vi "Generate Signal.vi"(11 "User Specified":T1={"Hardware Configuration"={"Signal Channel"="PXI1Slot7/ao0", "Response Channel"="PXI1Slot7/ai0", "Trigger Channel"="/PXI1Slot7/PFI0", "Number of Acquisitions"=1.0}, "Analysis Configuration"={"Statistics"=TRUE}, "Signal Type"=enum."From Excel", "New Data Behavior"=enum."Replace", "Signal Configuration"={"Chirp Amplitude"=0.0, "I/O Limit"=0.0, "Sample Rate"=0.0, "Chirp Duration (s)"=0.0, "Upper Frequency"=0.0, "Lower Frequency"=0.0, "Windowing"=enum."None"}, "Waveform File"="", "Save Location"=""}) -> (0 "Number of samples":dbl format="%0.2f", 1 "Y min":dbl format="%0.2f", 2 "Y max":dbl format="%0.2f", 3 "Final Waveform":waveform(dbl)(graph))   [LabVIEW 2017]
uses:
  controls/User Specified Data.ctl
  controls/HW Configuration.ctl
  controls/Analysis Configuration.ctl
  controls/New Data Behavior.ctl
  controls/Signal Configuration.ctl
  <vilib>/Waveform/WDTOps.llb/WDT Append Waveforms DBL.vi
  <vilib>/Waveform/WDTOps.llb/WDT Number of Waveform Samples DBL.vi
panel:
  out "Initial waveform":waveform(dbl)
  out "Shift register waveform":waveform(dbl)(graph)
  out "Number of rows":i32
  out "Voltage Offset":dbl
  out "Single Chirp w/ offset":waveform(dbl)(graph)
  out "Samples per chirp":dbl
  out "Single Chirp (Excel)":waveform(dbl)(graph)
  out "error out":errorcluster
  in  "error in":errorcluster
  # "D:\\Data\\7-02-2018\\SSPFM"
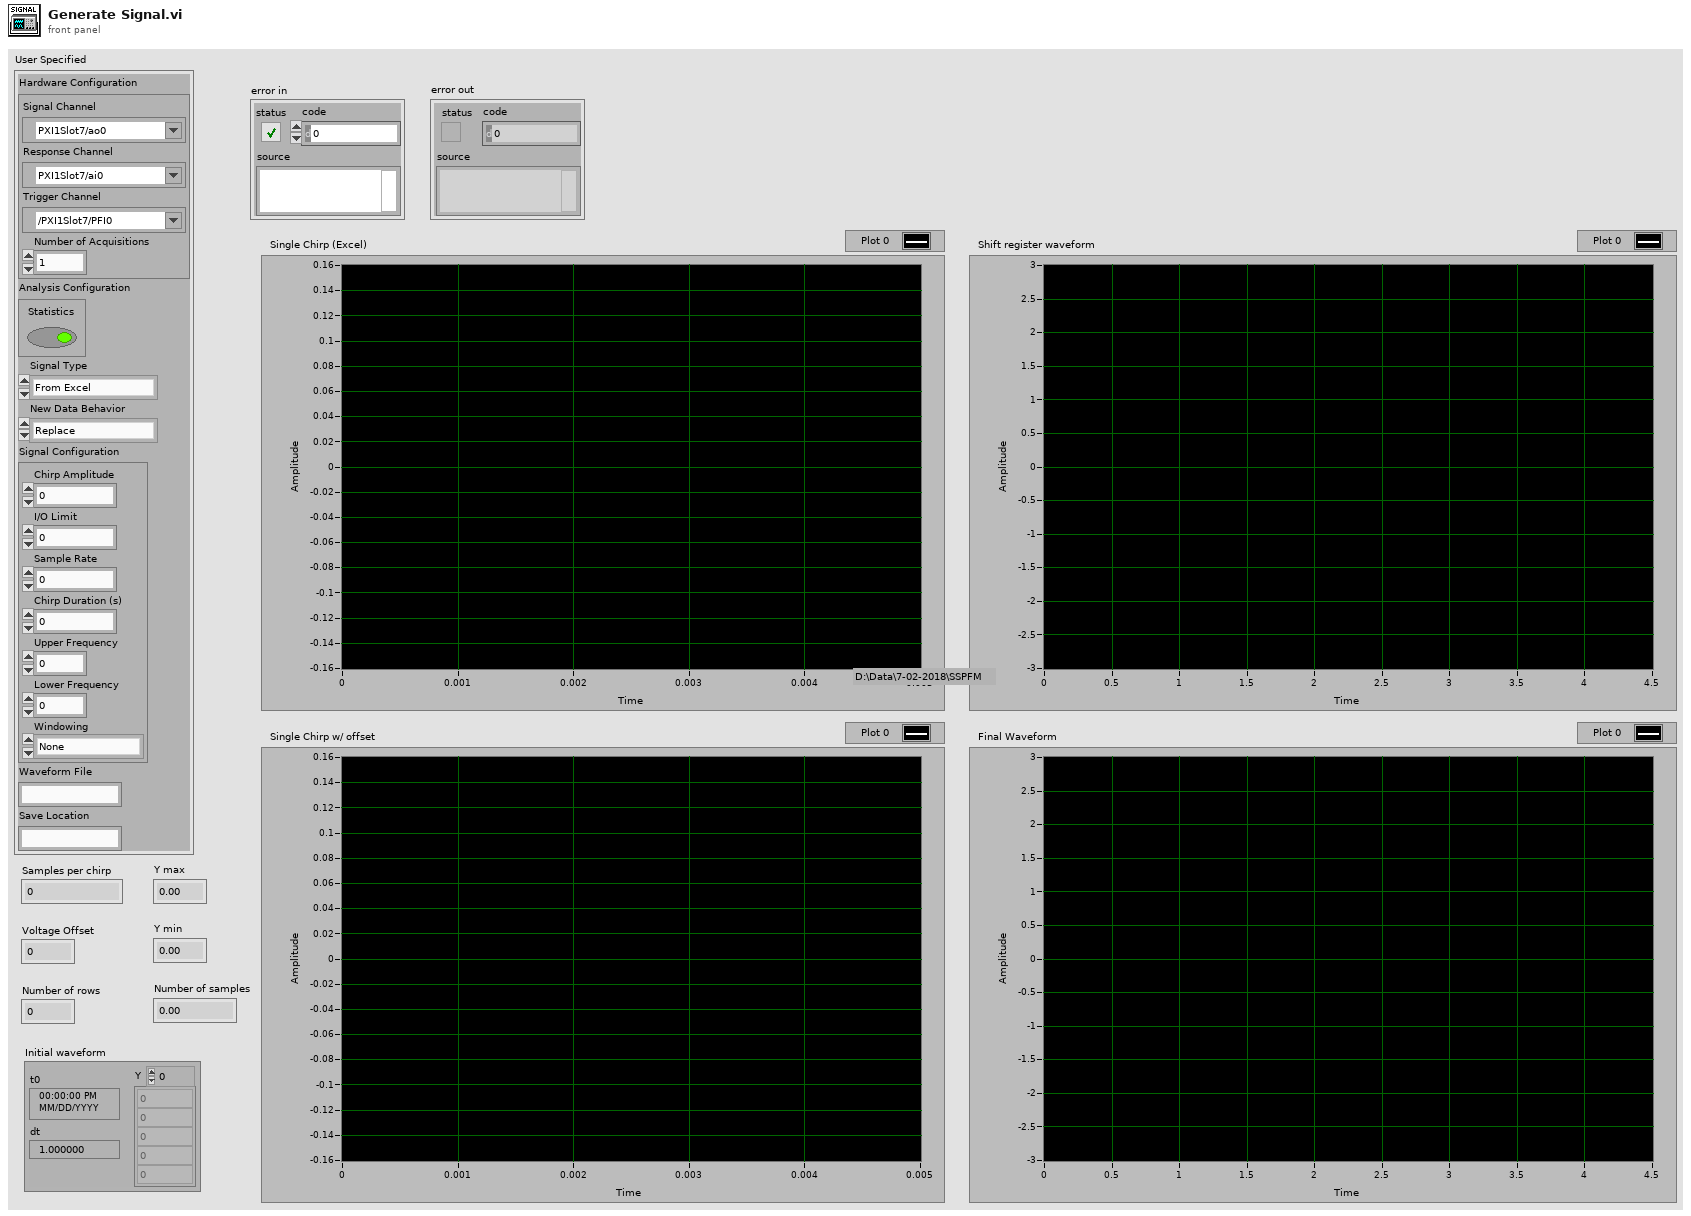
[diagram p1: front panel]
types:
  T1 = typedef "User Specified Data.ctl" = cluster{"Hardware Configuration":T2, "Analysis Configuration":T3, "Signal Type":enum16{"From Excel", "Single Chirp"}, "New Data Behavior":T4, "Signal Configuration":T5, "Waveform File":string, "Save Location":string}
  T2 = typedef "HW Configuration.ctl" = cluster{"Signal Channel":tag, "Response Channel":tag, "Trigger Channel":tag, "Number of Acquisitions":dbl}
  T3 = typedef "Analysis Configuration.ctl" = cluster{"Statistics":bool}
  T4 = typedef "New Data Behavior.ctl" = enum16{"Replace", "Overlay", "Append"}
  T5 = typedef "Signal Configuration.ctl" = cluster{"Chirp Amplitude":dbl, "I/O Limit":dbl, "Sample Rate":dbl, "Chirp Duration (s)":dbl, "Upper Frequency":dbl, "Lower Frequency":dbl, "Windowing":enum16{"None", "Exponential", "Flat top", "Hamming", "Hanning", "Kaiser-Bessel", "Rectangular"}}
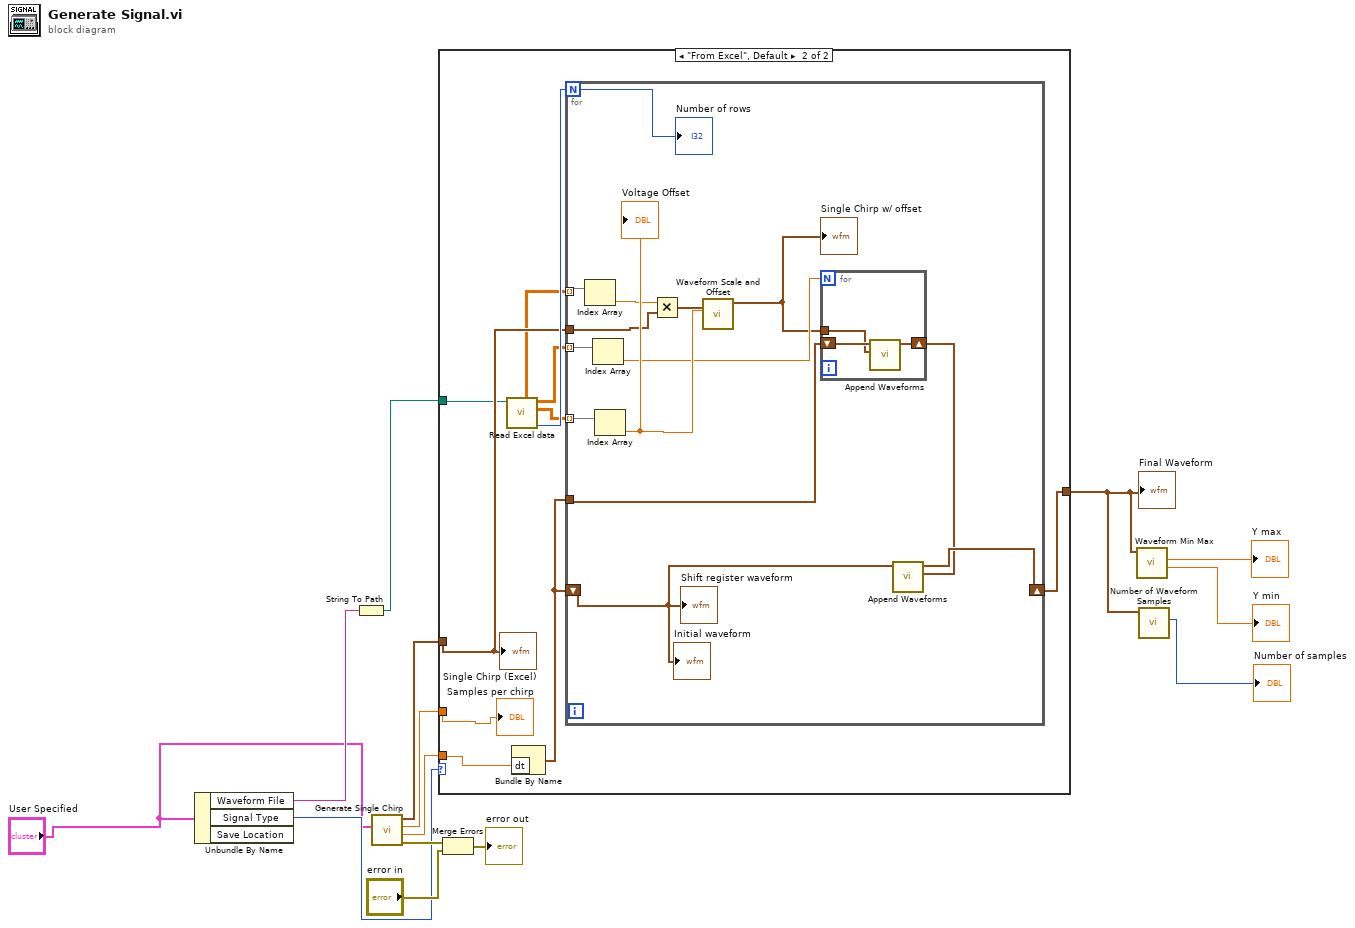
[diagram p0: block diagram]
diagram:
  n1 = Unbundle By Name("User Specified") -> ("Waveform File"=w3:string, "Signal Type"=w11:enum16{"From Excel", "Single Chirp"})  [unwired: 1 out]
  n2 = String To Path(string=w3) -> (path=w2:path)
  n3 = call "Generate Single Chirp.vi"("User Specified"="User Specified") -> ("error out"=w12:errorcluster, "dt"=w4:dbl, "Number of samples"=w10:dbl, "Chirp"=w9:waveform(dbl))  [unwired: 7 in]
  n4 = case shown="\"From Excel\", Default" w11 {
    tunnel: w9 -> [w15 w22]
    tunnel: w10 -> [_ w18]
    tunnel: w4 -> [_ w17]
    tunnel: [w15 w20] -> w6
    tunnel: w2 -> [_ w19]
    frame "Single Chirp" {
    }
    frame "From Excel", Default {
      n5 = call "Read Excel data.vi"("file path (dialog if empty)"=w19) -> ("Number of rows"=w25:i32, "Voltage Offsets"=w24:dbl[][], "Chirp Durations"=w23:dbl[][], "Multiplier"=w16:dbl[][])  [unwired: 7 in]
      n6 = Bundle By Name("dt"=w17) -> (w21:waveform(dbl))  [unwired: 1 in]
      n7 = for {
        N: w25 -> [w37]
        tunnel: w22 -> [w28]
        tunnel: w24 -> [w39] mode=indexing
        tunnel: w23 -> [w36] mode=indexing
        shift-right: [w35] -> w20
        shift-left: w21 -> [w34]
        tunnel: w21 -> [w32]
        tunnel: w16 -> [w30] mode=indexing
        n8 = Index Array(array=w30) -> (element=w29:dbl)  [unwired: 1 in]
        n9 = Index Array(array=w36) -> (element=w33:dbl)  [unwired: 1 in]
        n10 = Index Array(array=w39) -> (element=w38:dbl)  [unwired: 1 in]
        "Voltage Offset" <- w38
        n11 = Multiply(x=w29, y=w28) -> (x*y=w27:waveform(dbl))
        n12 = call <vilib>:"Waveform Scale and Offset.vi"("offset"=w38, "waveform in"=w27) -> ("waveform out"=w26:waveform(dbl))  [unwired: 8 in, 1 out]
        "Single Chirp w/ offset" <- w26
        n13 = for {
          N: w33 -> [_]
          tunnel: w26 -> [w41]
          shift-right: [w40] -> w31
          shift-left: w32 -> [w42]
          n14 = call-poly <vilib>:"Append Waveforms.vi"("waveform B"=w41, "waveform A"=w42) -> ("waveform out"=w40:waveform(dbl))  [unwired: 8 in, 1 out]
        }
        n15 = call-poly <vilib>:"Append Waveforms.vi"("waveform B"=w31, "waveform A"=w34) -> ("waveform out"=w35:waveform(dbl))  [unwired: 8 in, 1 out]
        "Number of rows" <- w37
        "Shift register waveform" <- w34
        "Initial waveform" <- w34
      }
      "Single Chirp (Excel)" <- w22
      "Samples per chirp" <- w18
    }
  }
  "Final Waveform" <- w6
  n16 = Merge Errors(w12, "error in") -> (→"error out":errorcluster)
  n17 = call <vilib>:"Waveform Min Max.vi"("waveform in"=w6) -> ("Y min"=→"Y min":dbl, "Y max"=→"Y max":dbl)  [unwired: 5 in, 4 out]
  n18 = call-poly <vilib>:"Number of Waveform Samples.vi"("waveform in"=w6) -> ("number of samples"=→"Number of samples":i32)  [unwired: 8 in, 2 out]
